vi "Disconnect from Server.vi"(8 "error in (no error)":errorcluster, 11 "Client in":refnum<class "Client.lvclass">) -> (0 "error out":errorcluster, 3 "Client out":refnum<class "Client.lvclass">)   [LabVIEW 2013, in "MQTT Server.lvlib" / "Client.lvclass"]
uses:
  Client.lvclass
  Client.lvclass/Client.ctl
  Connection/TCPConnection.lvclass
  Control Packets/DISCONNECT/DISCONNECT.lvclass
  Control Packets/ControlPacket/ControlPacket.lvclass
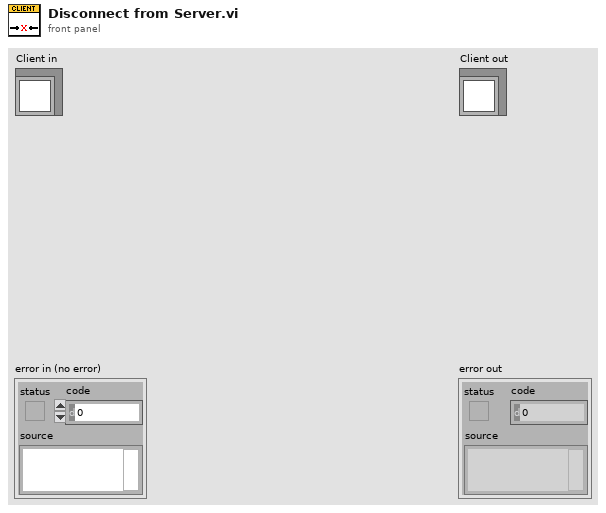
[diagram p1: front panel]
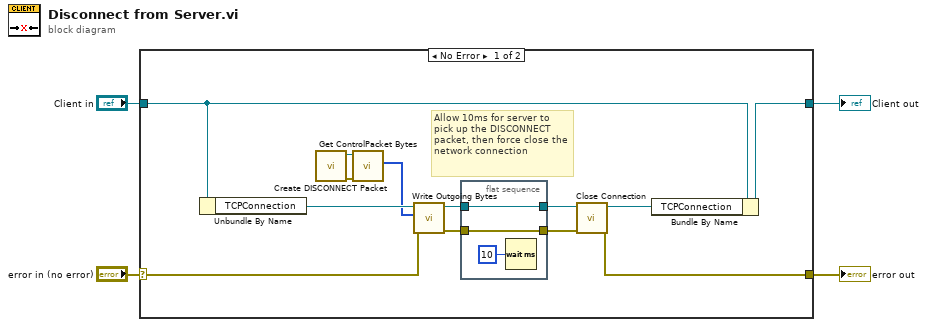
[diagram p0: block diagram]
diagram:
  n1 = case shown="No Error" "error in (no error)" {
    selector: "error in (no error)" -> [w14 w22]
    tunnel: [w5 w22] -> w3
    tunnel: [w17 w21] -> w1
    tunnel: "Client in" -> [w16 w21]
    frame No Error {
      # "Allow 10ms for server to pick up the DISCONNECT packet, then force close the  network connection"
      n2 = Unbundle By Name(w16) -> ("TCPConnection"=w15:refnum<class "TCPConnection.lvclass">)
      n3 = call "Create DISCONNECT Packet.vi"() -> ("error out"=w12:errorcluster, "DISCONNECT"=w13:refnum<class "DISCONNECT.lvclass">)  [unwired: 10 in]
      n4 = call "Get ControlPacket Bytes.vi"("error in (no error)"=w12, "ControlPacket"=w13) -> ("Bytes Stream"=w11:u8[])  [unwired: 7 in, 2 out]
      n5 = call "Write Outgoing Bytes.vi"("error in (no error)"=w14, "Bytes"=w11, "TCPConnection in"=w15) -> ("error out"=w7:errorcluster, "TCPConnection out"=w8:refnum<class "TCPConnection.lvclass">)  [unwired: 7 in]
      n6 = flat-sequence {
        tunnel: w8 -> [w20]
        tunnel: [w20] -> w9
        tunnel: [w18] -> w10
        tunnel: w7 -> [w18]
        frame #0 {
          n7 = Wait (ms)(milliseconds to wait=u32 10) -> ()  [unwired: 1 out]
        }
      }
      n8 = call-dynamic "Close Connection.vi"("error in (no error)"=w10, "TCPConnection in"=w9) -> ("error out"=w5:errorcluster, "TCPConnection out"=w6:refnum<class "TCPConnection.lvclass">)  [unwired: 8 in]
      n9 = Bundle By Name(cluster=w16, "TCPConnection"=w6) -> (w17:refnum<class "Client.lvclass">)
    }
    frame Error {
    }
  }
  "error out" <- w3
  "Client out" <- w1
